vi "1D Spring.vi"(7 "Parameters":T1={"Spring Stiffness"=0.1, "Deadzone Radius"=20.0}, 9 "desired pos":dbl, 10 "current pos":dbl) -> (2 "output":dbl)   [LabVIEW 2017, in "myPAM.lvlib"]
uses:
  myPAM.lvlib
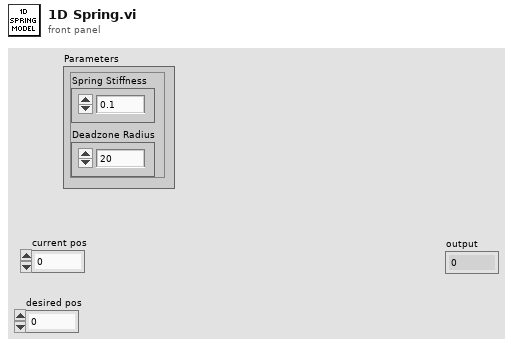
[diagram p1: front panel]
types:
  T1 = cluster{"Spring Stiffness":dbl, "Deadzone Radius":dbl}
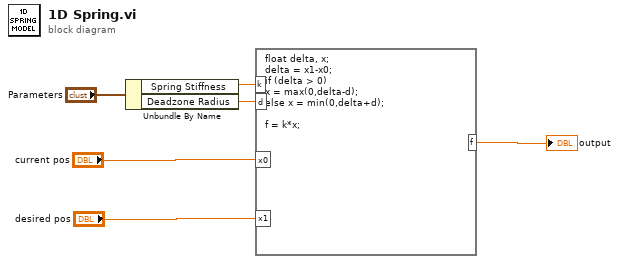
[diagram p0: block diagram]
diagram:
  n1 = Unbundle By Name("Parameters") -> ("Spring Stiffness"=w4:dbl, "Deadzone Radius"=w5:dbl)
  n2 = formula code="float delta, x;\ndelta = x1-x0;\nif (delta > 0)\nx = max(0,delta-d);\nelse x = min(0,delta+d);\n\nf = k*x;"("k"=w4, "d"=w5, "x0"="current pos", "x1"="desired pos") -> ("f"=→"output":dbl)
